vi "DisposeFaceEncoding.vi"(8 "error in (no error)":errorcluster, 11 "FaceEncoding in":refnum<k24>) -> (0 "error out":errorcluster)   [LabVIEW 2020]
uses:
  dll/FaceRecognitionDotNet.dll
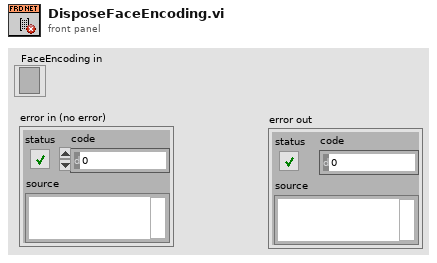
[diagram p1: front panel]
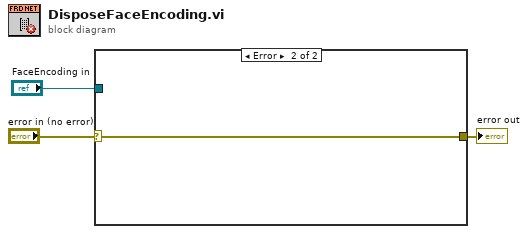
[diagram p0: block diagram]
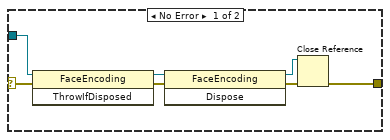
[diagram p2: hidden frame]
diagram:
  n1 = case shown="Error" "error in (no error)" {
    selector: "error in (no error)" -> [w5 w11]
    tunnel: "FaceEncoding in" -> [w6 _]
    tunnel: [w4 w11] -> w1
    frame No Error {
      n2 = invoke class="FaceEncoding" method="ThrowIfDisposed"(reference=w6, error in=w5) -> (reference out=w7:refnum<k24>, error out=w8:errorcluster)  [unwired: 1 in, 1 out]
      n3 = invoke class="FaceEncoding" method="Dispose"(reference=w7, error in=w8) -> (reference out=w9:refnum<k24>, error out=w10:errorcluster)  [unwired: 1 in, 1 out]
      n4 = Close Reference(reference=w9, error in (no error)=w10) -> (error out=w4:errorcluster)
    }
    frame Error {
    }
  }
  "error out" <- w1
